vi "Next_Core.vi"(8 "error in (no error)":errorcluster, 10 "Query Result in":refnum<class "DapperResult.lvclass">, 11 "SqlMapper in":refnum<class "SqlMapper.lvclass">) -> (0 "error out":errorcluster, 1 "Found":bool, 2 "Row as Variant":variant, 3 "SqlMapper out":refnum<class "SqlMapper.lvclass">)   [LabVIEW 2020, in "ORM_Dapper.lvlib" / "DapperResult.lvclass"]
uses:
  DapperResult.lvclass
  <vilib>/Viviota/shared/ORM.lvlibp/ORM/SqlMapper/SqlMapper.lvclass
  DapperResult.lvclass/DapperResult.ctl
  Read ref.vi
  DapperRow/DapperRow.lvclass
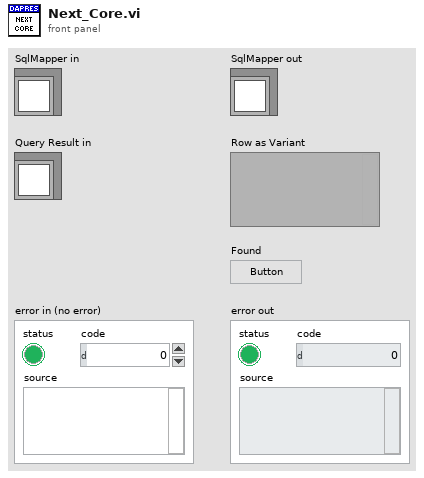
[diagram p1: front panel]
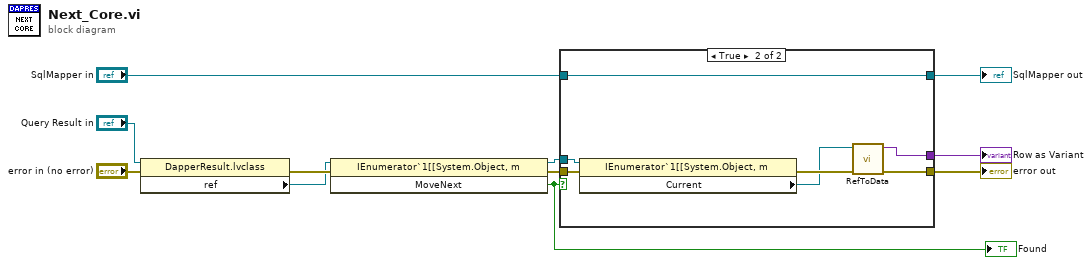
[diagram p0: block diagram]
diagram:
  n1 = property class="DapperResult.lvclass"(reference="Query Result in", error in="error in (no error)") -> (error out=w3:errorcluster, "ref"=w1:refnum<k24>)  [unwired: 1 out]
  n2 = invoke class="IEnumerator`1[[System.Object, m" method="MoveNext"(reference=w1, error in=w3) -> (reference out=w4:refnum<k24>, error out=w5:errorcluster, "MoveNext"=w9:bool)  [unwired: 1 in]
  "Found" <- w9
  n3 = case shown="True" w9 {
    tunnel: w4 -> [_ w20]
    tunnel: w5 -> [w13 w19]
    tunnel: [_ w14] -> w6
    tunnel: [w13 w16] -> w7
    tunnel: [w12 w18] -> w10
    tunnel: "SqlMapper in" -> [w12 w18]
    frame False {
    }
    frame True {
      n4 = property class="IEnumerator`1[[System.Object, m"(reference=w20, error in=w19) -> (error out=w17:errorcluster, "Current"=w15:refnum<k24>)  [unwired: 1 out]
      n5 = call "RefToData.vi"("error in (no error)"=w17, ".NET Refnum in"=w15) -> ("error out"=w16:errorcluster, "variant out"=w14:variant)  [unwired: 8 in]
    }
  }
  "SqlMapper out" <- w10
  "error out" <- w7
  "Row as Variant" <- w6
